vi "roll rate_angle(SubVI).vi"(11 "Roll Rate/angle [deg]":dbl[](array[numeric])) -> (2 "Roll Angle[rad]":dbl[](array[numeric]), 3 "Roll Rate[rad/s]":dbl[](array[numeric]))   [LabVIEW 2017]
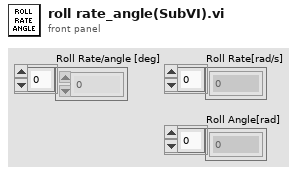
[diagram p1: front panel]
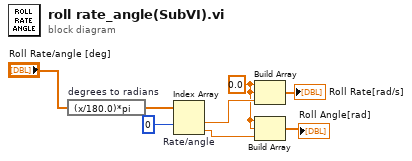
[diagram p0: block diagram]
diagram:
  w4 = 0.0 ("element")
  n1 = expression code="(x/180.0)*pi" "degrees to radians"("Roll Rate/angle [deg]") -> (w2:dbl[])
  n2 = Index Array "Rate/angle"(array=w2, index #1=0 ("index")) -> (element #1=w5:dbl, element #2=w6:dbl)  [unwired: 1 in]
  n3 = Build Array(w4, w4, w5) -> (→"Roll Rate[rad/s]":dbl[])
  n4 = Build Array(w4, w4, w6) -> (→"Roll Angle[rad]":dbl[])
